vi "LighthouseFinal.vi"(0 "Image In":T1) -> (1 "Image Out":T1, 2 "output cluster":cluster{"Pos. X":i32, "Pos. Y":i32})   [LabVIEW 2014]
uses:
  <vilib>/vision/Image Controls.llb/IMAQ Image.ctl
  <vilib>/vision/NI_Vision_Development_Module.lvlib
panel:
  out "error out":errorcluster
  in  "error in":errorcluster
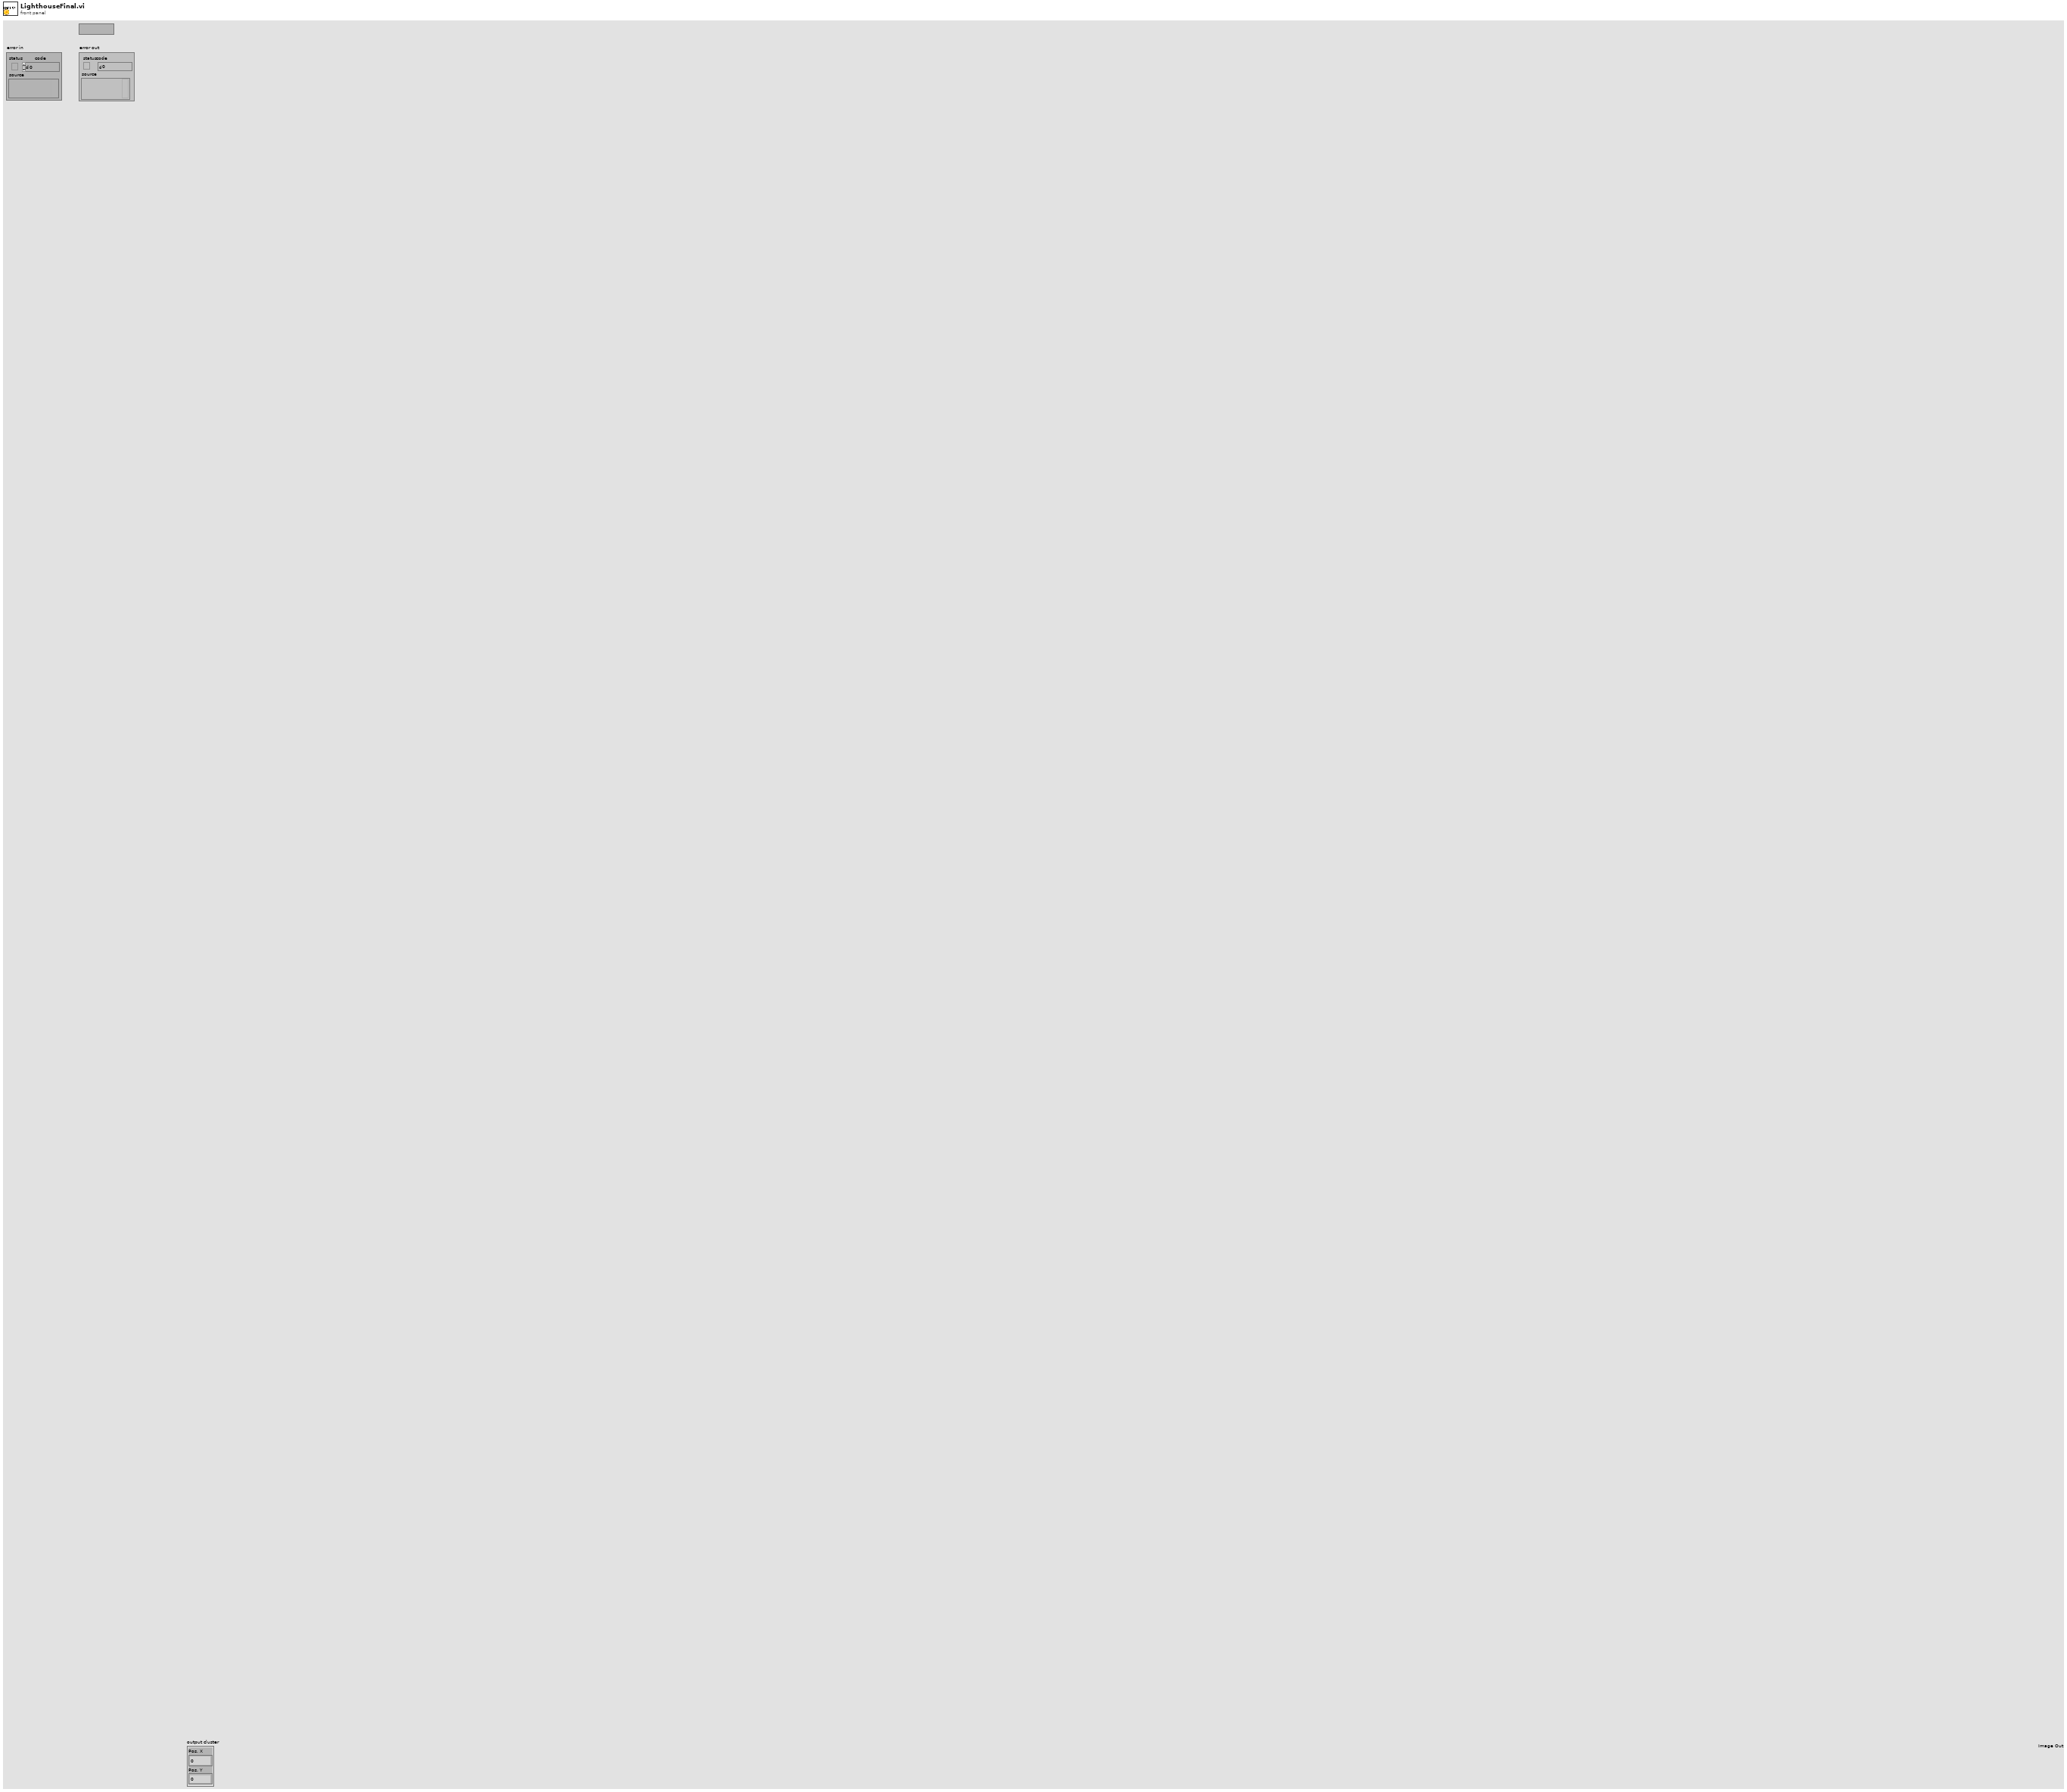
[diagram p1: front panel]
types:
  T1 = typedef "IMAQ Image.ctl" = refnum<image>
  T2 = cluster{"Measurement Parameter":i32, "Range Lower Value":dbl, "Range Upper Value":dbl, "Range":bool, "Measurement Type":bool}[]
  T3 = enum32{"AutoM", "Close", "Dilate", "Erode", "Gradient", "Gradient out", "Gradient in", "Hit miss", "Open", "PClose", "POpen", "Thick", "Thin"}
  T4 = typedef "Image Type" = u32
  T5 = cluster{"Global Rectangle":i32[], "Contours":cluster{"ID":enum32{"External", "Internal"}, "Type":u32, "Coordinates":i32[]}[]}
  T6 = cluster{"Pos. X":i32, "Pos. Y":i32, "Radius":i32, "Core Area":i32}[]
  T7 = cluster{"Pos. X":i32, "Pos. Y":i32, "Radius":i32, "Core Area":i32}
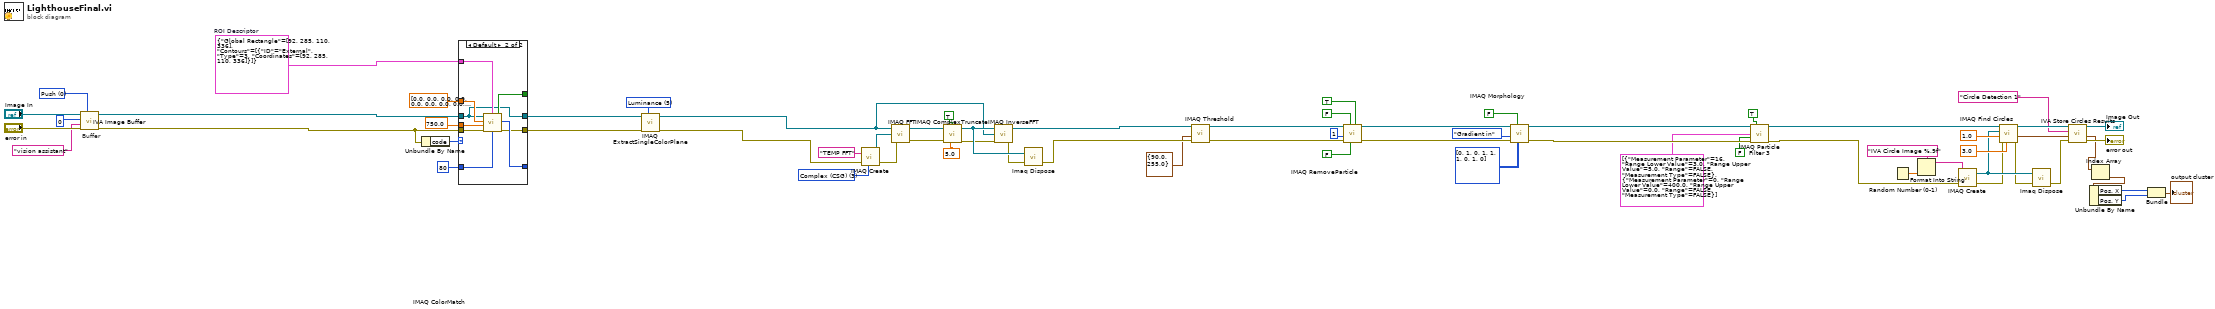
[diagram p0: block diagram]
diagram:
  w39 = T4 3 items=["Grayscale (U8)", "Grayscale (I16)", "Grayscale (SGL)", "Complex (CSG)", "RGB (U32)", "HSL (U32)", "RGB (U64)", "Grayscale (U16)"] ("Image Type")
  w54 = 5 items=["Red", "Green", "Blue", "Hue", "Saturation", "Luminance", "Value", "Intensity"] ("Color Plane")
  w56 = T5 {"Global Rectangle"=[92, 285, 110, 336], "Contours"=[{"ID"=enum."External", "Type"=3, "Coordinates"=[92, 285, 110, 336]}]}  # ROI Descriptor
  w64 = u16 0 items=["Push", "Pop", "Reset"] ("Function")
  # "Buffer"
  n1 = call <vilib>:"IVA Image Buffer.vi"("Function"=w64, "error in (no error)"="error in", "Prefix"="vision assistant", "Buffer #"=0, "Image In"="Image In") -> ("error out"=w65:errorcluster, "Image Out"=w58:T1)  [unwired: 5 out]
  n2 = Unbundle By Name(w65) -> ("code"=w55:i32)
  n3 = case shown="Default" w55 {
    tunnel: 750.0 ("Minimum Match Score") -> [_ w77]
    tunnel: 80 ("Match Saturation Threshold") -> [_ w76]
    tunnel: dbl[] [0.0, 0.0, 0.0, 0.0, 0.0, 0.0, 0.0, 0.0, 0.011574074074074073, 0.0, 0.26851851851851855, 0.0, 0.6458333333333334, 0.0, 0.07407407407407407, 0.0, 0.0, 0.0, 0.0, 0.0, 0.0, 0.0, 0.0, 0.0, 0.0, 0.0, 0.0, 0.0, 0.0, 0.0, 0.0, 0.0, 0.0, 0.0, 0.0, 0.0, 0.0, 0.0, 0.0, 0.0, 0.0, 0.0, 0.0, 0.0, 0.0, 0.0, 0.0, 0.0, 0.0, 0.0, 0.0, 0.0, 0.0, 0.0, 0.0, 0.0, 0.0, 0.0] ("Color Spectrum") -> [_ w75]
    tunnel: [_ w74] -> _
    tunnel: [_ w73] -> _
    tunnel: w58 -> [w68 w69]
    tunnel: w65 -> [_ w72]
    tunnel: [_ w71] -> w57
    tunnel: w56 -> [_ w70]
    tunnel: [w68 w69] -> w53
    frame -1074396199, -1074396198 {
      # "Discard\nCoordinate\nSystem Error"
    }
    frame Default {
      n4 = call "IMAQ ColorMatch"("ROI Descriptor"=w70, "Image"=w69, "Color Spectrum"=w75, "Match Saturation Threshold"=w76, "Minimum Match Score"=w77, "error in (no error)"=w72) -> ("Match Flag"=w74:bool[], "Match Score"=w73:i32[], "error out"=w71:errorcluster)  [unwired: 1 out]
    }
  }
  n5 = call "IMAQ ExtractSingleColorPlane"("Color Plane"=w54, "error in (no error)"=w57, "Image Src"=w53) -> ("error out"=w52:errorcluster, "Image Dst Out"=w42:T1)  [unwired: 1 in, 6 out]
  n6 = call "IMAQ Create"("Image Name"="TEMP FFT", "Image Type"=w39, "error in (no error)"=w52) -> ("New Image"=w50:T1, "error out"=w43:errorcluster)  [unwired: 1 in, 1 out]
  n7 = call "IMAQ FFT"("error in (no error)"=w43, "Image Dst"=w50, "Image Src"=w42) -> ("error out"=w48:errorcluster, "Image Dst Out"=w49:T1)  [unwired: 1 out]
  n8 = call "IMAQ ComplexTruncate"("error in (no error)"=w48, "Truncation Frequency %"=sgl 5.0, "Image Src"=w49, "Low pass/High pass (Low pass)"=TRUE) -> ("error out"=w46:errorcluster, "Image Dst Out"=w47:T1)  [unwired: 1 in, 2 out]
  n9 = call "IMAQ InverseFFT"("error in (no error)"=w46, "Image Dst"=w42, "Image Src"=w47) -> ("error out"=w45:errorcluster, "Image Dst Out"=w37:T1)  [unwired: 1 out]
  n10 = call "Imaq Dispose"("Image"=w47, "error in (no error)"=w45) -> ("error out"=w44:errorcluster)  [unwired: 1 in, 3 out]
  n11 = call "IMAQ Threshold"("error in (no error)"=w44, "Range"=cluster{"Lower value":sgl, "Upper value":sgl} {"Lower value"=90.0, "Upper value"=255.0}, "Image Src"=w37) -> ("error out"=w36:errorcluster, "Image Dst Out"=w31:T1)  [unwired: 3 in, 4 out]
  n12 = call "IMAQ RemoveParticle"("Connectivity 4/8 (8)"=TRUE, "Low Pass/High Pass (Low)"=FALSE, "Square/Hexa (Square)"=FALSE, "error in (no error)"=w36, "Number of Erosion"=1, "Image Src"=w31) -> ("error out"=w30:errorcluster, "Image Dst Out"=w26:T1)  [unwired: 1 in, 3 out]
  n13 = call "IMAQ Morphology"("Structuring Element"=i32[][] [[0, 1, 0], [1, 1, 1], [0, 1, 0]], "Square/Hexa (Square)"=FALSE, "error in (no error)"=w30, "Operation"=T3."Gradient in", "Image Src"=w26) -> ("error out"=w25:errorcluster, "Image Dst Out"=w21:T1)  [unwired: 2 in, 3 out]
  n14 = call "IMAQ Particle Filter 3"("Image Src"=w21, "Connectivity 4/8 (8)"=TRUE, "Selection Values"=T2 [{"Measurement Parameter"=16, "Range Lower Value"=3.0, "Range Upper Value"=5.0, "Range"=FALSE, "Measurement Type"=FALSE}, {"Measurement Parameter"=0, "Range Lower Value"=400.0, "Range Upper Value"=0.0, "Range"=FALSE, "Measurement Type"=FALSE}], "Keep/Remove Particles (F)"=FALSE ("Keep/Remove Particles"), "error in (no error)"=w25) -> ("Image Dst Out"=w12:T1, "error out"=w22:errorcluster)  [unwired: 4 in, 5 out]
  n15 = Random Number (0-1)() -> (number: 0 to 1=w6:dbl)
  n16 = Format Into String(format string="IVA Circle Image %.9f" ("Image Name"), w6) -> (resulting string=w8:string)  [unwired: 2 in, 1 out]
  n17 = call "IMAQ Create"("Image Name"=w8, "error in (no error)"=w22) -> ("New Image"=w17:T1, "error out"=w16:errorcluster)  [unwired: 2 in, 1 out]
  n18 = call "IMAQ Find Circles"("Max Radius"=sgl 3.0, "error in (no error)"=w16, "Min Radius"=sgl 1.0, "Image Dst"=w17, "Image Src"=w12) -> ("error out"=w15:errorcluster, "Circles Data"=w9:T6)  [unwired: 5 out]
  n19 = call "Imaq Dispose"("Image"=w17, "error in (no error)"=w15) -> ("error out"=w14:errorcluster)  [unwired: 1 in, 3 out]
  n20 = call <vilib>:"IVA Store Circles Results.vi"("error in (no error)"=w14, "Circles Data"=w9, "Step Name"="Circle Detection 1", "Image in"=w12) -> ("error out"=→"error out":errorcluster, "Circles Data (calibrated)"=w2:T6, "Image dup"=→"Image Out":T1)  [unwired: 5 out]
  n21 = Index Array(array=w2) -> (element=w5:T7)  [unwired: 1 in]
  n22 = Unbundle By Name(w5) -> ("Pos. X"=w4:i32, "Pos. Y"=w3:i32)
  n23 = Bundle("Pos. X"=w4, "Pos. Y"=w3) -> (→"output cluster":cluster{"Pos. X":i32, "Pos. Y":i32})  [unwired: 1 in]
